vi "CalcDesiredTorque-FromCable.vi"(8 "error in (no error)":errorcluster, 11 "CAlexData2 in":refnum<class "CAlexData2.lvclass">) -> (0 "error out":errorcluster, 2 "Joint Torque Des":dbl[][](array[numeric]), 3 "CAlexData2 out":refnum<class "CAlexData2.lvclass">)   [LabVIEW 2014]
uses:
  ExpData/ExpData.lvclass
  CableSerialChain/CableSerialChain.lvclass
  CAlexData2.lvclass
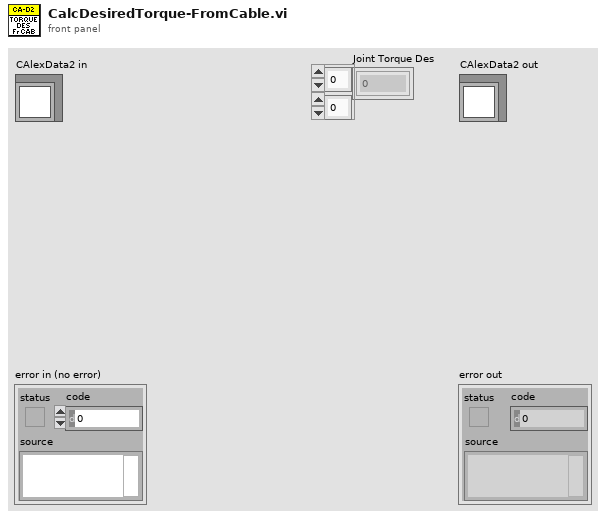
[diagram p1: front panel]
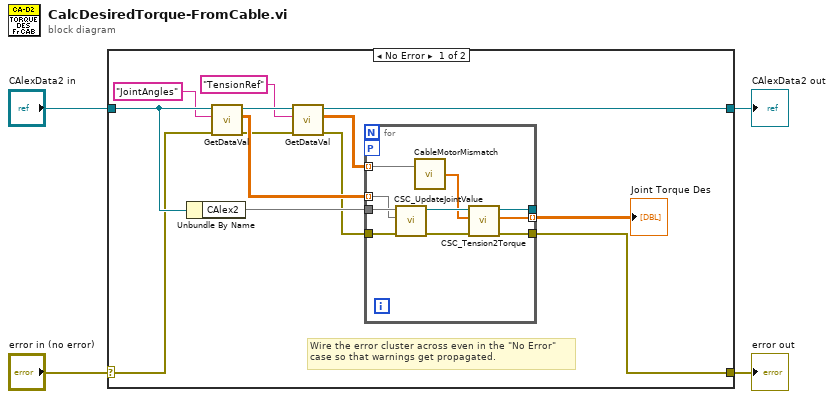
[diagram p0: block diagram]
diagram:
  n1 = case shown="No Error" "error in (no error)" {
    selector: "error in (no error)" -> [w7 w29]
    tunnel: [w5 w29] -> w3
    tunnel: [w12 w28] -> w1
    tunnel: "CAlexData2 in" -> [w16 w28]
    frame No Error {
      # "Wire the error cluster across even in the \"No Error\"\ncase so that warnings get propagated."
      n2 = Unbundle By Name(w16) -> ("CAlex2"=w15)
      n3 = call "GetDataVal.vi"("error in (no error)"=w7, "Name"="JointAngles", "CarexMData in"=w16) -> ("error out"=w8:errorcluster, "Data"=w11:dbl[][], "CarexMData out"=w17:refnum<class "CAlexData2.lvclass">)  [unwired: 5 in, 1 out]
      n4 = call "GetDataVal.vi"("error in (no error)"=w8, "Name"="TensionRef", "CarexMData in"=w17) -> ("error out"=w6:errorcluster, "Data"=w10:dbl[][], "CarexMData out"=w12:refnum<class "CAlexData2.lvclass">)  [unwired: 5 in, 1 out]
      n5 = for {
        tunnel: w11 -> [w26] mode=indexing
        tunnel: w10 -> [w19] mode=indexing
        tunnel: [w23] -> w9 mode=indexing
        workers-P: _ -> [_]
        tunnel: w15 -> [w27]
        tunnel: [w22] -> _
        tunnel: w6 -> [w21]
        tunnel: [w20] -> w5
        n6 = call "CSC_UpdateJointValue.vi"("error in (no error)"=w21, "JointValue (rad|m)"=w26, "C-Alex in"=w27) -> ("error out"=w24:errorcluster, "C-Alex out"=w25:refnum<class "CableSerialChain.lvclass">)  [unwired: 7 in]
        n7 = call "CableMotorMismatch.vi"("MotorTension"=w19) -> ("CableTension"=w18:dbl[])  [unwired: 2 in]
        n8 = call-dynamic "CSC_Tension2Torque.vi"("error in (no error)"=w24, "Cable Tensions"=w18, "CSC in"=w25) -> ("error out"=w20:errorcluster, "Joint Torque"=w23:dbl[], "CSC out"=w22:refnum<class "CableSerialChain.lvclass">)  [unwired: 6 in]
      }
      "Joint Torque Des" <- w9
    }
    frame Error {
    }
  }
  "error out" <- w3
  "CAlexData2 out" <- w1
